vi "Datalogger v3.vi"(8 "error in":errorcluster, 9 "1D data":string[](array[string]), 10 "append to file? (new file:F)":bool, 11 "file path (dialog if empty)":path) -> (0 "error out":errorcluster, 3 "path":path)   [LabVIEW 2012]
panel:
  in  "prompt":string
  in  "format (%s)":string="%s"
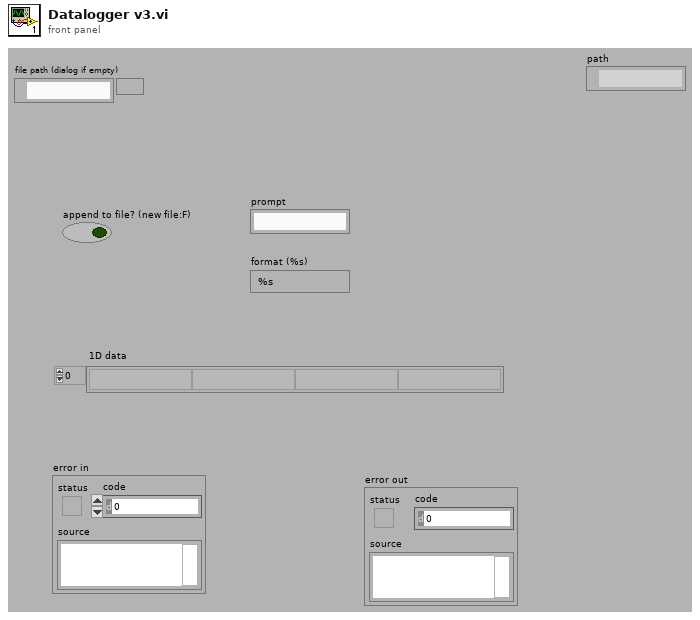
[diagram p1: front panel]
types:
  T1 = enum16{"open", "replace", "create", "open or create", "replace or create", "replace or create with confirmation"}
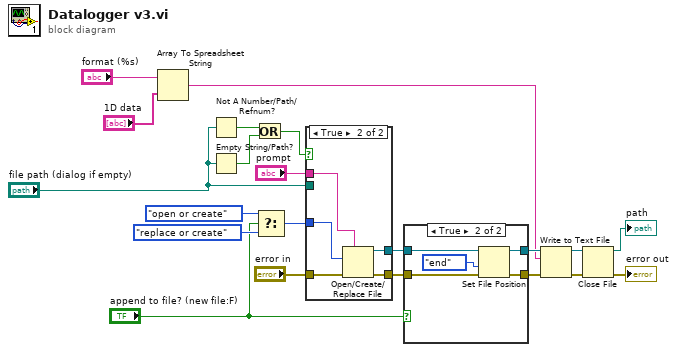
[diagram p0: block diagram]
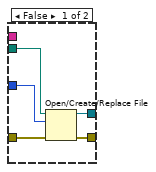
[diagram p3: hidden frame]
diagram:
  n1 = Array To Spreadsheet String(array="1D data", 3:"format (%s)") -> (spreadsheet string=w1:string)  [unwired: 1 in]
  n2 = Not A Number/Path/Refnum?(number/path/refnum="file path (dialog if empty)") -> (NaN/Path/Refnum?=w12:bool)
  n3 = Empty String/Path?(string/path="file path (dialog if empty)") -> (empty?=w13:bool)
  n4 = Or(x=w12, y=w13) -> (x .or. y?=w11:bool)
  n5 = Select ("function")(t=T1."open or create" ("operation (0:open)"), s="append to file? (new file:F)", f=T1."replace or create" ("operation (0:open)")) -> (s? t:f=w7:T1)
  n6 = case shown="True" w11 {
    tunnel: "prompt" -> [_ w29]
    tunnel: "error in" -> [w26 w30]
    tunnel: [w25 w31] -> w5
    tunnel: [w24 w28] -> w4
    tunnel: "file path (dialog if empty)" -> [w23 _]
    tunnel: w7 -> [w22 w27]
    frame False {
      n7 = Open/Create/Replace File(file path (use dialog)=w23, error in=w26, operation (0:open)=w22) -> (refnum out=w24:refnum<file>, error out=w25:errorcluster)  [unwired: 3 in, 1 out]
    }
    frame True {
      n8 = Open/Create/Replace File(error in=w30, prompt=w29, operation (0:open)=w27) -> (refnum out=w28:refnum<file>, error out=w31:errorcluster)  [unwired: 3 in, 1 out]
    }
  }
  n9 = case shown="True" "append to file? (new file:F)" {
    tunnel: w5 -> [w32 w38]
    tunnel: [w32 w37] -> w6
    tunnel: w4 -> [w33 w35]
    tunnel: [w33 w36] -> w3
    frame False {
    }
    frame True {
      n10 = Set File Position(refnum=w35, from (0:start)=enum16{"start", "end", "current"}."end", error in=w38) -> (refnum out=w36:refnum<file>, error out=w37:errorcluster)  [unwired: 1 in]
    }
  }
  n11 = Write to Text File(file (use dialog)=w3, text=w1, error in=w6) -> (refnum out=w15:refnum<file>, error out=w14:errorcluster)  [unwired: 1 in, 1 out]
  n12 = Close File(refnum=w15, error in=w14) -> (path=→"path":path, error out=→"error out":errorcluster)
